vi "Q&L PLC&5U TCP Read-Write-Code.vi"(0 "Read/Write":bool, 1 "Devices":enum16{"B", "W", "M", "D"}(ring), 5 "Command":T1(ring), 7 "Address":string="001000", 9 "Devices Count":string="0A00", 11 "Write Data":string[](array[string]), 12 "Write":string) -> (4 "Data Out":string)   [LabVIEW 2014]
panel:
  in  "Write Data1":string="01000200"
  in  "Byte Length":string="0026"
  # "Read Bit:       0401\nRead Word:   0400\nWrite Bit:       1401\nWrite Word:   1400"
  # "B:A0\nW:B4\nM:90\nD:A8"
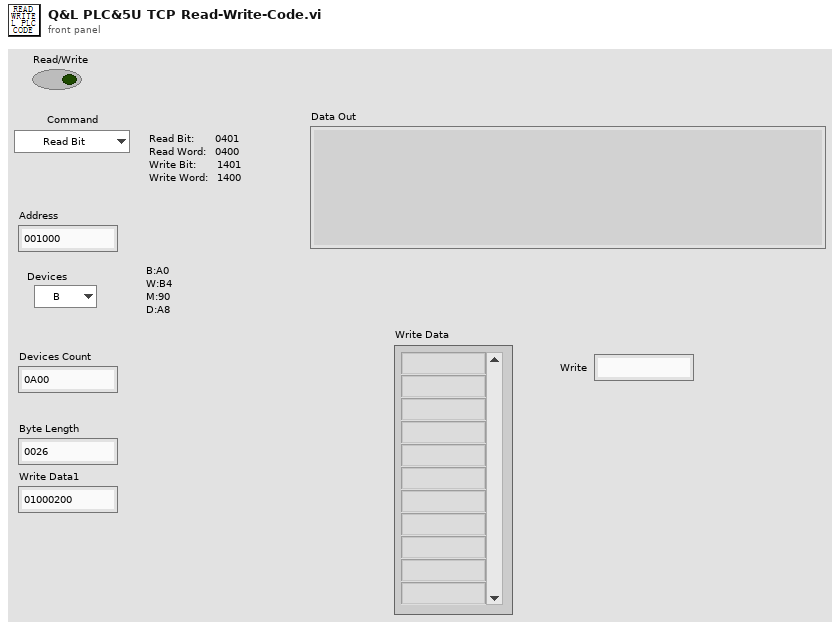
[diagram p1: front panel]
types:
  T1 = enum16{"Read Bit", "Read Word", "Write Bit", "Write Word"}
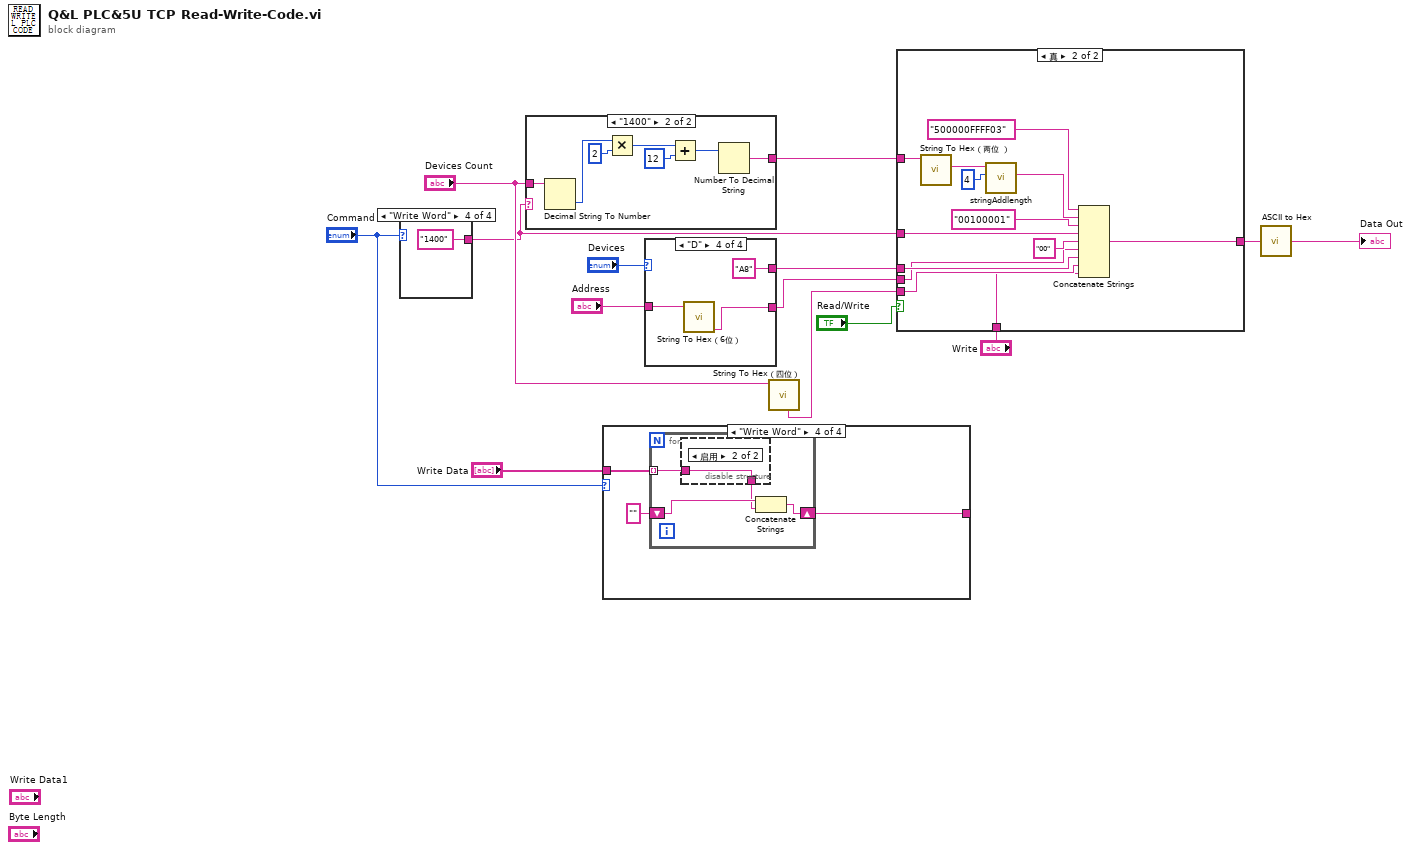
[diagram p0: block diagram]
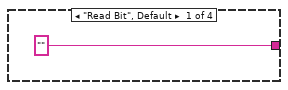
[diagram p2: hidden frame]
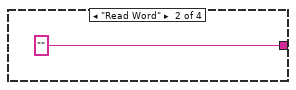
[diagram p3: hidden frame]
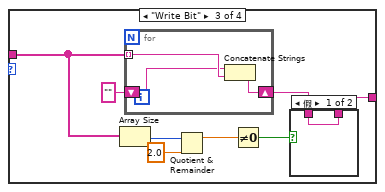
[diagram p4: hidden frame]
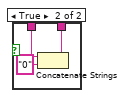
[diagram p5: hidden frame]
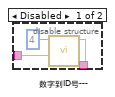
[diagram p6: hidden frame]
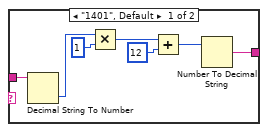
[diagram p7: hidden frame]
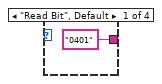
[diagram p8: hidden frame]
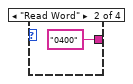
[diagram p9: hidden frame]
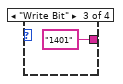
[diagram p10: hidden frame]
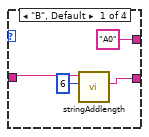
[diagram p11: hidden frame]
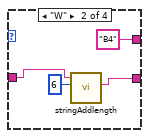
[diagram p12: hidden frame]
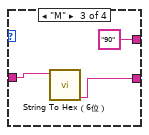
[diagram p13: hidden frame]
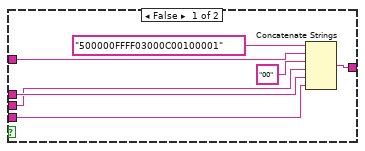
[diagram p14: hidden frame]
diagram:
  n1 = case shown="\"Write Word\"" "Command" {
    tunnel: ["0401" "0400" "1401" "1400"] -> w8
    frame "Read Bit", Default {
    }
    frame "Read Word" {
    }
    frame "Write Bit" {
    }
    frame "Write Word" {
    }
  }
  n2 = case shown="\"1400\"" w8 {
    tunnel: "Devices Count" -> [w20 w32]
    tunnel: [w19 w26] -> w7
    frame "1401", Default {
      n3 = Decimal String To Number(string=w20) -> (number=w25:i32)  [unwired: 2 in, 1 out]
      n4 = Multiply(x=w25, y=1) -> (x*y=w23:i32)
      n5 = Add(x=w23, y=12) -> (x+y=w21:i32)
      n6 = Number To Decimal String(number=w21) -> (decimal integer string=w19:string)  [unwired: 1 in]
    }
    frame "1400" {
      n7 = Decimal String To Number(string=w32) -> (number=w31:i32)  [unwired: 2 in, 1 out]
      n8 = Multiply(x=w31, y=2) -> (x*y=w29:i32)
      n9 = Add(x=w29, y=12) -> (x+y=w27:i32)
      n10 = Number To Decimal String(number=w27) -> (decimal integer string=w26:string)  [unwired: 1 in]
    }
  }
  n11 = case shown="\"Write Word\"" "Command" {
    tunnel: "Write Data" -> [_ _ w42 w52]
    tunnel: ["" "" w36 w51] -> _
    frame "Read Bit", Default {
    }
    frame "Read Word" {
    }
    frame "Write Bit" {
      n12 = Array Size(array=w42) -> (size(s)=w41:i32)
      n13 = for {
        tunnel: w42 -> [w49] mode=indexing
        shift-right: [w47] -> w38
        shift-left: "" -> [w48]
        n14 = Concatenate Strings(w48, w49) -> (w47:string)
      }
      n15 = Quotient & Remainder(x=w41, y=2.0) -> (x-y*floor(x/y)=w39:dbl)  [unwired: 1 out]
      n16 = Not Equal To 0?(x=w39) -> (x != 0?=w37:bool)
      n17 = case shown="假" w37 {
        tunnel: w38 -> [w43 w45]
        tunnel: [w43 w44] -> w36
        frame False {
        }
        frame True {
          n18 = Concatenate Strings(w45, "0" ("字符串")) -> (w44:string)
        }
      }
    }
    frame "Write Word" {
      n19 = for {
        tunnel: w52 -> [w56] mode=indexing
        shift-right: [w55] -> w51
        shift-left: "" -> [w54]
        n20 = disable-structure shown="启用" {
          disable-tunnel: w56 -> [w59 w60]
          disable-tunnel: [w57 w60] -> w53
          frame Disabled {
            n21 = call "数字到ID号---.vi"("字符串"=w59, "个数"=4) -> ("子字符串"=w57:string)  [unwired: 5 in, 4 out]
          }
          frame Enabled {
          }
        }
        n22 = Concatenate Strings(w54, w53) -> (w55:string)
      }
    }
  }
  n23 = case shown="\"D\"" "Devices" {
    tunnel: ["A0" "B4" "90" "A8"] -> w11
    tunnel: "Address" -> [w62 w65 w69 w73]
    tunnel: [w63 w66 w70 w72] -> w5
    frame "B", Default {
      n24 = call "stringAddlength.vi"("length"=6, "Input"=w62) -> ("Out"=w63:string)  [unwired: 8 in, 1 out]
    }
    frame "W" {
      n25 = call "stringAddlength.vi"("length"=6, "Input"=w65) -> ("Out"=w66:string)  [unwired: 8 in, 1 out]
    }
    frame "M" {
      n26 = call "String To Hex（6位）.vi"("String"=w69) -> ("高低对调数据"=w70:string)  [unwired: 7 in, 3 out]
    }
    frame "D" {
      n27 = call "String To Hex（6位）.vi"("String"=w73) -> ("高低对调数据"=w72:string)  [unwired: 7 in, 3 out]
    }
  }
  n28 = call "String To Hex（四位）.vi"("String"="Devices Count") -> ("连接的字符串"=w1:string)  [unwired: 6 in, 4 out]
  n29 = case shown="真" "Read/Write" {
    tunnel: w8 -> [w80 w91]
    tunnel: w5 -> [w75 w83]
    tunnel: [w78 w93] -> w14
    tunnel: w11 -> [w77 w89]
    tunnel: w1 -> [w76 w90]
    tunnel: w7 -> [_ w86]
    tunnel: "Write" -> [_ w82]
    frame False {
      n30 = Concatenate Strings("500000FFFF03000C00100001" ("字符串"), w80, "00" ("字符串"), w75, w77, w76) -> (w78:string)
    }
    frame True {
      n31 = call "String To Hex（两位 ）.vi"("String"=w86) -> ("Out"=w85:string)  [unwired: 9 in, 1 out]
      n32 = call "stringAddlength.vi"("length"=4, "Input"=w85) -> ("Out"=w87:string)  [unwired: 8 in, 1 out]
      n33 = Concatenate Strings("500000FFFF03" ("字符串"), w87, "00100001" ("字符串"), w91, "00" ("字符串"), w83, w89, w90, w82) -> (w93:string)
    }
  }
  n34 = call "ASCII to Hex.vi"("ASCII"=w14) -> ("Hex"=→"Data Out":string)
